vi "Contain.vi"(8 "error in (no error)":errorcluster caption="错误输入（无错误）", 10 "Item":variant, 11 "Queue 输入":refnum<class "Queue.lvclass"> caption="DNL_LabVIEW Object in") -> (0 "error out":errorcluster caption="错误输出", 2 "Contains":bool, 3 "Queue 输出":refnum<class "Queue.lvclass"> caption="DNL_LabVIEW Object out")   [LabVIEW 2012, in "Queue.lvclass"]
uses:
  Queue.lvclass
  Queue.lvclass/Queue.ctl
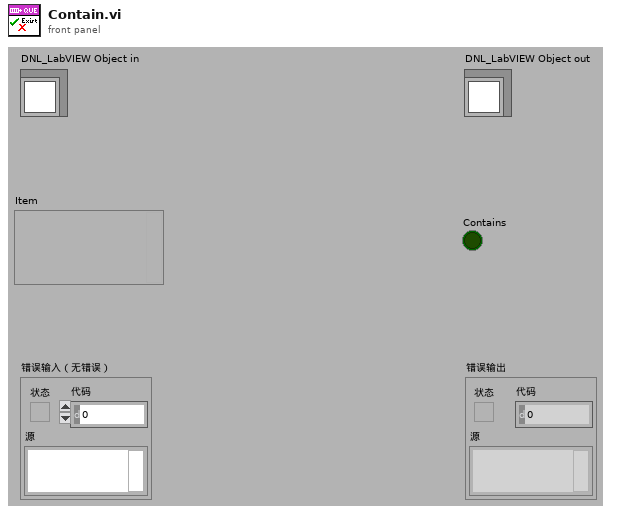
[diagram p1: front panel]
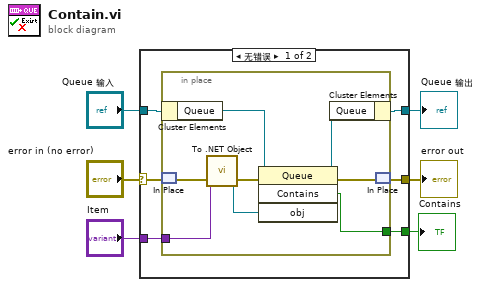
[diagram p0: block diagram]
diagram:
  n1 = case shown="无错误" "error in (no error)" {
    selector: "error in (no error)" -> [w10 w22]
    tunnel: [w9 w22] -> w5
    tunnel: [w11 w21] -> w3
    tunnel: "Queue 输入" -> [w12 w21]
    tunnel: "Item" -> [w8 _]
    tunnel: [w7 _] -> w1
    frame No Error {
      n2 = in-place {
        in-place-border: w8 -> [w14]
        in-place-border: [w13] -> w7
        n3 = in-place-cluster #1(w12) -> ("Queue"=w20:refnum<k24>)
        n4 = in-place-match #2(w10) -> (w16:errorcluster)
        n5 = call <vilib>:"To .NET Object.vi"("error in (no error)"=w16, "anything"=w14) -> ("error out"=w15:errorcluster, ".NET object"=w17:refnum<k24>)
        n6 = invoke class="Queue" method="Contains"(reference=w20, error in=w15, "obj"=w17) -> (reference out=w19:refnum<k24>, error out=w18:errorcluster, "Contains"=w13:bool)  [unwired: 1 in, 1 out]
        n7 = in-place-cluster #1("Queue"=w19) -> (w11:refnum<class "Queue.lvclass">)
        n8 = in-place-match #2(w18) -> (w9:errorcluster)
      }
    }
    frame Error {
    }
  }
  "error out" <- w5
  "Queue 输出" <- w3
  "Contains" <- w1
